vi "Add CIPC Error.vi"(8 "error in (no error)":errorcluster, 9 "String to Append":string, 10 "Error":T1, 11 "Insert Error":bool=TRUE) -> (0 "error out":errorcluster)   [LabVIEW 2021, in "CIF_NI_CIPC.lvlib"]
uses:
  CIF_NI_CIPC.lvlib
  <vilib>/CIF Foundation/CIF Utilities/Errors/Errors_CIF_U.lvlib
  TypeDefs/Errors.ctl
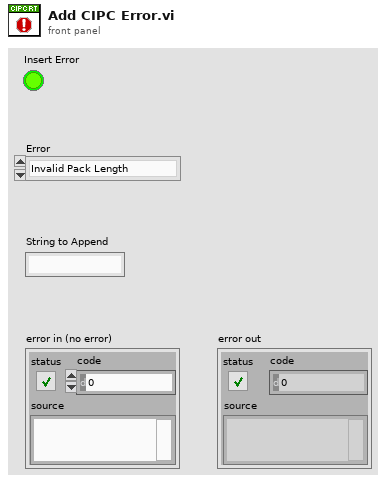
[diagram p1: front panel]
types:
  T1 = typedef "CIF_NI_CIPC.lvlib/Errors.ctl" = enum16{"Invalid Pack Length", "Invalid Pack Destination", "Unsupported Type", "Missing Library"}
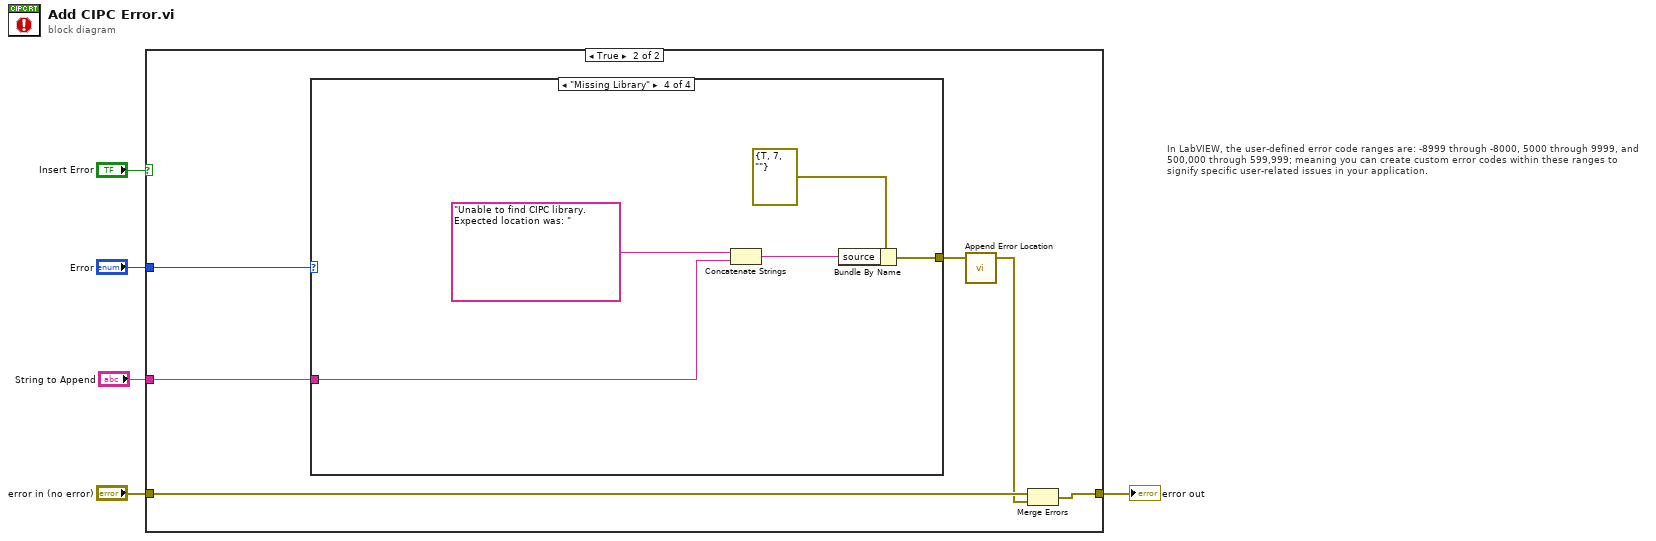
[diagram p0: block diagram]
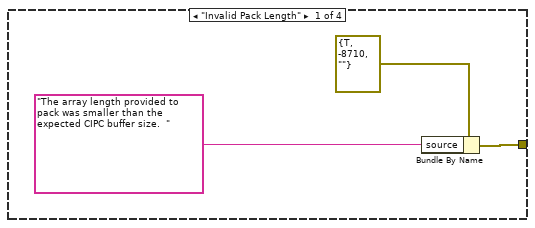
[diagram p3: hidden frame]
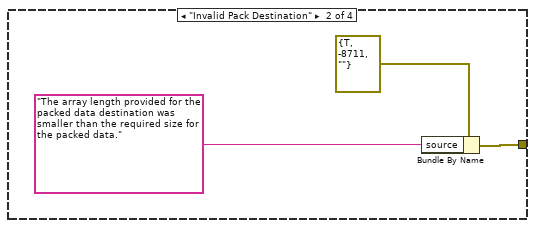
[diagram p4: hidden frame]
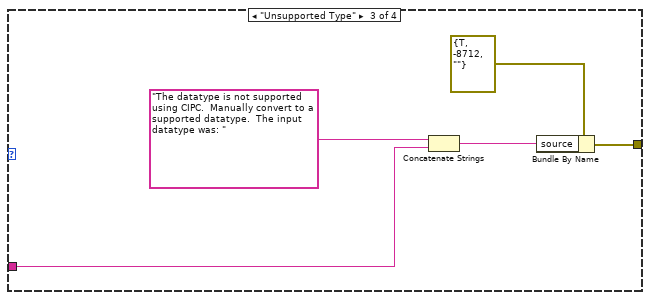
[diagram p5: hidden frame]
diagram:
  # "In LabVIEW, the user-defined error code ranges are: -8999 through -8000, 5000 through 9999, and 500,000 through 599,999; meaning you can create custom error codes within these ranges to signify specific user-related issues in your application."
  n1 = case shown="True" "Insert Error" {
    tunnel: [w6 w9] -> w4
    tunnel: "error in (no error)" -> [w6 w10]
    tunnel: "Error" -> [_ w12]
    tunnel: "String to Append" -> [_ w11]
    frame False {
    }
    frame True {
      n2 = case shown="\"Missing Library\"" w12 {
        tunnel: w11 -> [_ _ w19 w24]
        tunnel: [w14 w17 w22 w27] -> w8
        frame "Invalid Pack Length" {
          n3 = Bundle By Name(cluster=errorcluster {"status"=TRUE, "code"=-8710, "source"=""} ("Invalid ID"), "source"="The array length provided to pack was smaller than the expected CIPC buffer size.  ") -> (w14:errorcluster)
        }
        frame "Invalid Pack Destination" {
          n4 = Bundle By Name(cluster=errorcluster {"status"=TRUE, "code"=-8711, "source"=""} ("Invalid ID"), "source"="The array length provided for the packed data destination was smaller than the required size for the packed data.") -> (w17:errorcluster)
        }
        frame "Unsupported Type" {
          n5 = Concatenate Strings("The datatype is not supported using CIPC.  Manually convert to a supported datatype.  The input datatype was: " ("source"), w19) -> (w20:string)
          n6 = Bundle By Name(cluster=errorcluster {"status"=TRUE, "code"=-8712, "source"=""} ("Invalid ID"), "source"=w20) -> (w22:errorcluster)
        }
        frame "Missing Library" {
          n7 = Concatenate Strings("Unable to find CIPC library.  Expected location was: " ("source"), w24) -> (w25:string)
          n8 = Bundle By Name(cluster=errorcluster {"status"=TRUE, "code"=7, "source"=""} ("Invalid ID"), "source"=w25) -> (w27:errorcluster)
        }
      }
      n9 = call <vilib>:"Append Error Location.vi"("error in (no error)"=w8) -> ("error out"=w7:errorcluster)  [unwired: 4 in]
      n10 = Merge Errors(w10, w7) -> (w9:errorcluster)
    }
  }
  "error out" <- w4
